vi "Access Orient3d.vi"(7 "Get/Set":enum16{"Get", "Set"}(ring), 8 "error in (no error)":errorcluster, 9 "Value in":refnum<class "Orient3d Class.lvclass">, 10 "Key":string, 11 "FlexWorktable in":refnum<class "FlexWorktable.lvclass">) -> (0 "error out":errorcluster, 1 "Value out":refnum<class "Orient3d Class.lvclass">, 3 "FlexWorktable out":refnum<class "FlexWorktable.lvclass">)   [LabVIEW 2017, in "FlexWorktable.lvclass"]
uses:
  FlexWorktable.lvclass
  Orient3d Class/Orient3d Class.lvclass
  FlexWorktable.lvclass/FlexWorktable.ctl
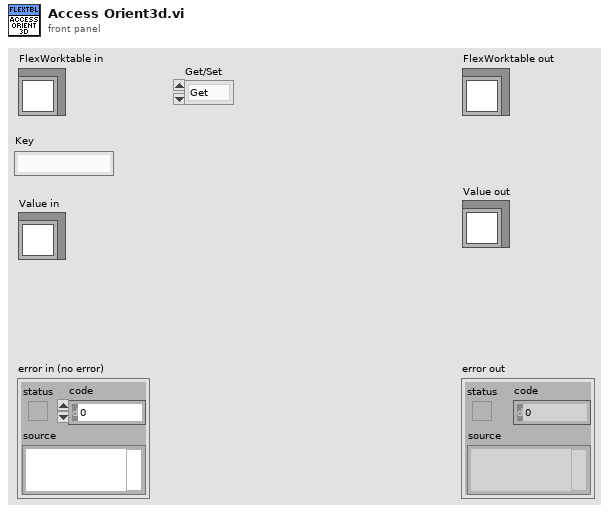
[diagram p1: front panel]
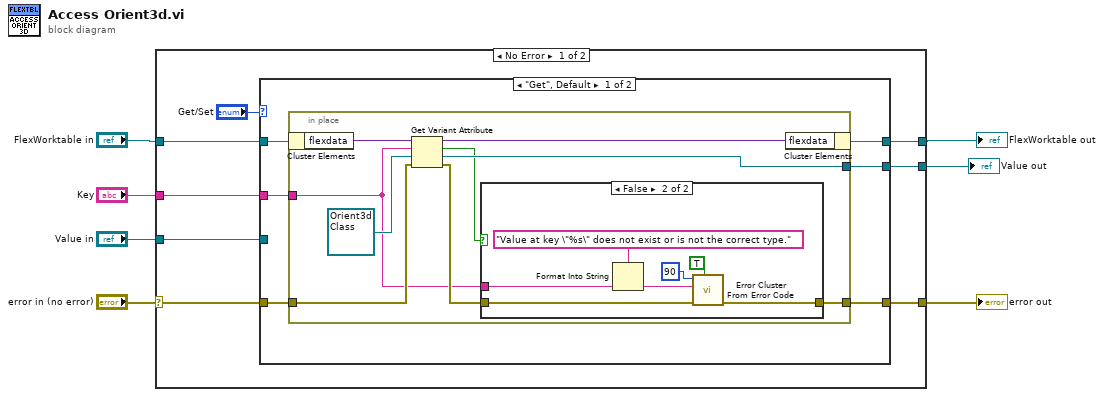
[diagram p0: block diagram]
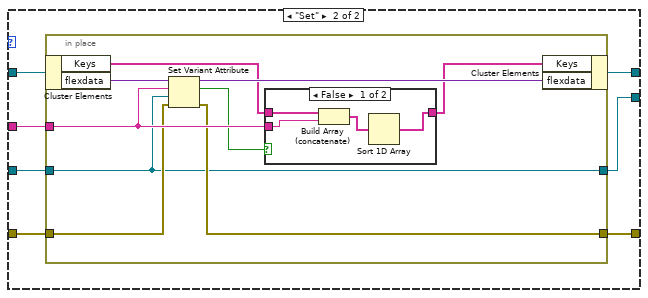
[diagram p3: hidden frame]
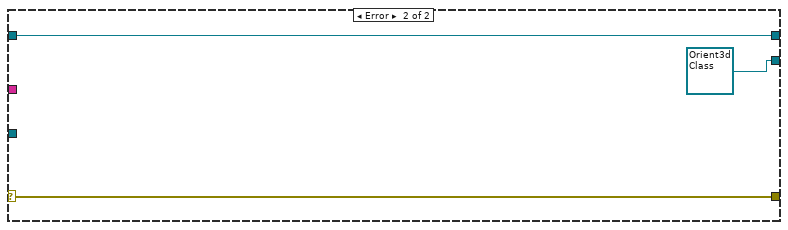
[diagram p5: hidden frame]
diagram:
  n1 = case shown="No Error" "error in (no error)" {
    selector: "error in (no error)" -> [w14 w62]
    tunnel: [w11 w62] -> w5
    tunnel: [w10 w61] -> w6
    tunnel: "FlexWorktable in" -> [w15 w61]
    tunnel: "Key" -> [w13 _]
    tunnel: "Value in" -> [w12 _]
    tunnel: [w8 refnum<class "Orient3d Class.lvclass"> refnum ("Orient3d Class.lvclass")] -> w1
    frame No Error {
      n2 = case shown="\"Get\", Default" "Get/Set" {
        tunnel: w15 -> [w21 w45]
        tunnel: w14 -> [w19 w44]
        tunnel: w13 -> [w20 w43]
        tunnel: w12 -> [_ w42]
        tunnel: [w17 w41] -> w11
        tunnel: [w18 w40] -> w10
        tunnel: [w16 w39] -> w8
        frame "Get", Default {
          n3 = in-place {
            in-place-border: w19 -> [w28]
            in-place-border: w20 -> [w23]
            in-place-border: [w25] -> w17
            in-place-border: [w27] -> w16
            n4 = in-place-cluster #1(w21) -> ("flexdata"=w30:variant)
            n5 = Get Variant Attribute(Variant=w30, name=w23, default value (empty Variant)=refnum<class "Orient3d Class.lvclass"> refnum ("Orient3d Class.lvclass"), error in=w28) -> (duplicate Variant=w29:variant, found=w22:bool, value=w27:refnum<class "Orient3d Class.lvclass">, error out=w24:errorcluster)
            n6 = case shown="False" w22 {
              tunnel: w23 -> [_ w35]
              tunnel: w24 -> [w31 w34]
              tunnel: [w31 w33] -> w25
              frame True {
              }
              frame False {
                n7 = Format Into String(format string="Value at key \"%s\" does not exist or is not the correct type.", w35) -> (resulting string=w36:string)  [unwired: 2 in, 1 out]
                n8 = call <vilib>:"Error Cluster From Error Code.vi"("show call chain? (False)"=TRUE, "error in (no error)"=w34, "error message (\"\")"=w36, "error code (0)"=90) -> ("error out"=w33:errorcluster)  [unwired: 5 in]
              }
            }
            n9 = in-place-cluster #1("flexdata"=w29) -> (w18:refnum<class "FlexWorktable.lvclass">)
          }
        }
        frame "Set" {
          n10 = in-place {
            in-place-border: w44 -> [w50]
            in-place-border: w43 -> [w51]
            in-place-border: w42 -> [w46]
            in-place-border: [w49] -> w41
            in-place-border: [w46] -> w39
            n11 = in-place-cluster #2(w45) -> ("Keys"=w52:string[], "flexdata"=w54:variant)
            n12 = Set Variant Attribute(Variant=w54, name=w51, value=w46, error in=w50) -> (Variant out=w53:variant, replaced=w48:bool, error out=w49:errorcluster)
            n13 = case shown="False" w48 {
              tunnel: w52 -> [w58 w59]
              tunnel: w51 -> [w57 _]
              tunnel: [w55 w59] -> w47
              frame False {
                n14 = Build Array (concatenate)(w58, w57) -> (w56:string[])
                n15 = Sort 1D Array(array=w56) -> (sorted array=w55:string[])
              }
              frame True {
              }
            }
            n16 = in-place-cluster #2("Keys"=w47, "flexdata"=w53) -> (w40:refnum<class "FlexWorktable.lvclass">)
          }
        }
      }
    }
    frame Error {
    }
  }
  "error out" <- w5
  "FlexWorktable out" <- w6
  "Value out" <- w1
